vi "Reset Output Protection.vi"(8 "error in (no error)":errorcluster, 11 "VISA resource name":refnum<visa-resource-name>) -> (0 "error out":errorcluster, 3 "VISA resource name out":refnum<visa-resource-name>)   [LabVIEW 2012, in "BK Precision 913XX.lvlib"]
doc: "Resets the status of over voltage protection (OVP)."
uses:
  <instrlib>/BK Precision 913XX/BK Precision 913XX.lvlib
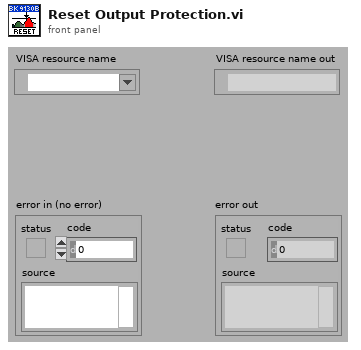
[diagram p1: front panel]
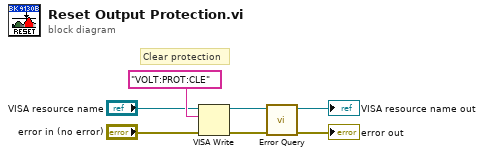
[diagram p0: block diagram]
diagram:
  # "Clear protection"
  n1 = VISA Write(VISA resource name="VISA resource name", write buffer="VOLT:PROT:CLE", error in (no error)="error in (no error)") -> (VISA resource name out=w5:refnum<visa-resource-name>, error out=w7:errorcluster)  [unwired: 1 out]
  n2 = call <instrlib>:"Error Query.vi"("error in (no error)"=w7, "VISA resource name"=w5) -> ("error out"=→"error out":errorcluster, "VISA resource name out"=→"VISA resource name out":refnum<visa-resource-name>)  [unwired: 6 in, 2 out]
